vi "File_Set Path to Keeper.vi"(7 "INI File Path":path, 8 "Error":errorcluster, 9 "Path To Set":path, 11 "File / Directory Name":string) -> (0 "Error Out":errorcluster, 2 "Valid Item Out":bool, 3 "Path Out":path=path "D:/Pitney PTS/PTS PROGRAMS/2-Sparks 1 and 2/SparksMain32.vi")   [LabVIEW 2020]
uses:
  <vilib>/Utility/config.llb/NI_LVConfig.lvlib
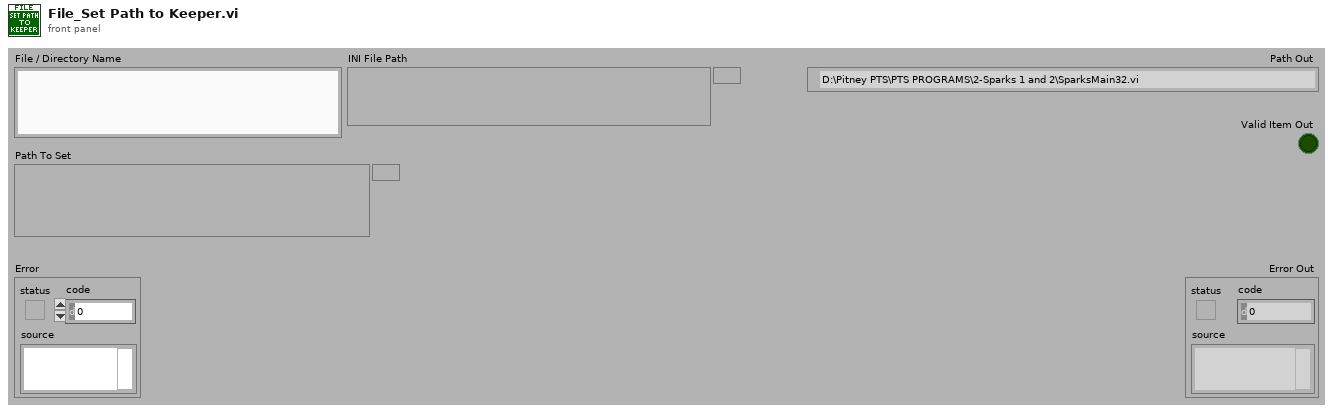
[diagram p1: front panel]
types:
  T1 = typedef "NI_LVConfig.lvlib/Config Data RefNum.ctl" = refnum<k1>
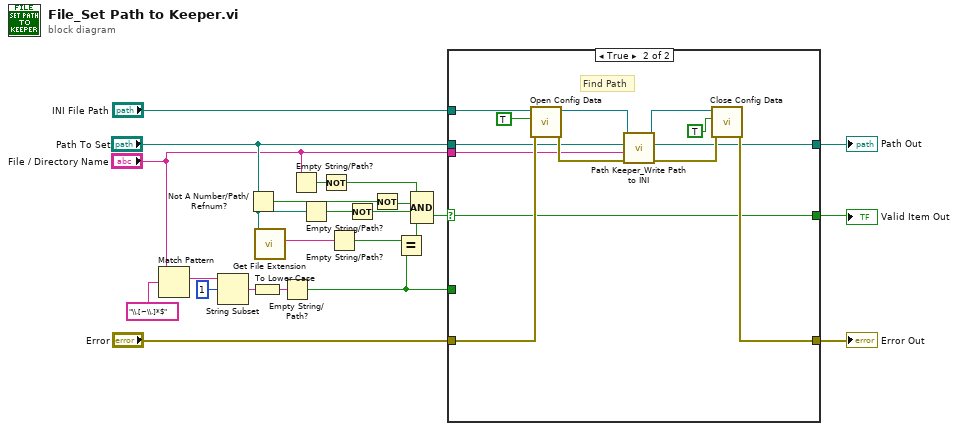
[diagram p0: block diagram]
diagram:
  n1 = Match Pattern(string="File / Directory Name", regular expression="\\.[~\\.]*$") -> (match substring=w10:string)  [unwired: 4 out]
  n2 = String Subset(string=w10, offset (0)=1) -> (substring=w9:string)  [unwired: 1 out]
  n3 = Not A Number/Path/Refnum?(number/path/refnum="Path To Set") -> (NaN/Path/Refnum?=w16:bool)
  n4 = To Lower Case(string=w9) -> (all lower case string=w6:string)
  n5 = call <vilib>:"Get File Extension.vi"("file"="Path To Set") -> ("lowercase file extension"=w12:string)  [unwired: 6 in, 4 out]
  n6 = Empty String/Path?(string/path=w6) -> (empty?=w5:bool)
  n7 = Empty String/Path?(string/path="File / Directory Name") -> (empty?=w4:bool)
  n8 = Empty String/Path?(string/path="Path To Set") -> (empty?=w18:bool)
  n9 = Not(x=w4) -> (.not. x?=w2:bool)
  n10 = Empty String/Path?(string/path=w12) -> (empty?=w11:bool)
  n11 = Not(x=w18) -> (.not. x?=w17:bool)
  n12 = Not(x=w16) -> (.not. x?=w15:bool)
  n13 = Equal?(x=w11, y=w5) -> (x = y?=w19:bool)
  n14 = Compound Arithmetic op=AND(w2, w15, w17, w19) -> (w1:bool)
  n15 = case shown="True" w1 {
    selector: w1 -> [w24 w28]
    tunnel: [w26 w39] -> w22
    tunnel: "Error" -> [w26 w35]
    tunnel: [w25 w29] -> w20
    tunnel: [w24 w28] -> w21
    tunnel: "INI File Path" -> [_ w37]
    tunnel: "File / Directory Name" -> [_ w27]
    tunnel: w5 -> [_ _]
    tunnel: "Path To Set" -> [w25 w30]
    frame False {
    }
    frame True {
      # "Find Path"
      n16 = call <vilib>:"Open Config Data.vi"("error in (no error)"=w35, "create file if necessary (T)"=TRUE ("create file if necessary? (T)"), "configuration file path"=w37) -> ("error out"=w32:errorcluster, "refnum"=w34:T1)  [unwired: 6 in, 1 out]
      n17 = call "Path Keeper_Write Path to INI.vi"("Error In"=w32, "File / Directory Name In"=w27, "Path In"=w30, "Ini Ref In"=w34) -> ("Error Out"=w31:errorcluster, "Path Out"=w29:path, "Ini Ref Out"=w33:T1)  [unwired: 5 in]
      n18 = call <vilib>:"Close Config Data.vi"("error in (no error)"=w31, "write file if changed (T)"=TRUE, "refnum"=w33) -> ("error out"=w39:errorcluster)  [unwired: 7 in, 1 out]
    }
  }
  "Path Out" <- w20
  "Error Out" <- w22
  "Valid Item Out" <- w21
